vi "readFromXML.vi"(8 "error in (no error)":errorcluster, 10 "XMLin":string, 11 "RADecTarget in":refnum<class "RADecTarget.lvclass">) -> (0 "error out":errorcluster, 3 "RADecTarget out":refnum<class "RADecTarget.lvclass">)   [LabVIEW 2014, in "TCSDataDefinitions.lvlib" / "TCSCommand.lvlib" / "TargetConfiguration.lvlib" / "Target.lvlib" / "FixedTarget.lvlib" / "RADecTarget.lvclass"]
uses:
  RADecTarget.lvclass
  RADecTarget.lvclass/RADecTarget.ctl
  FixedTarget/FixedTarget.lvclass
  RADecParameters/RADecParameters.lvclass
  <userlib>/Common/XML/XMLParser/XMLParser.lvclass
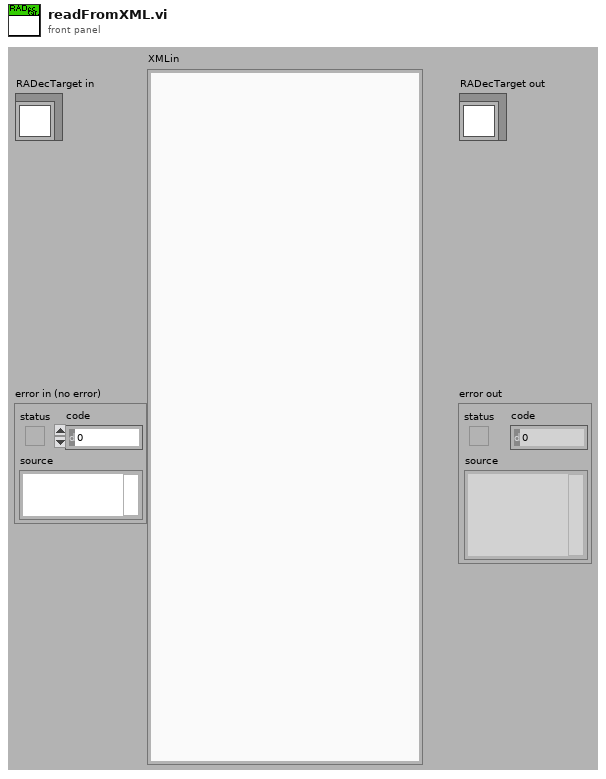
[diagram p1: front panel]
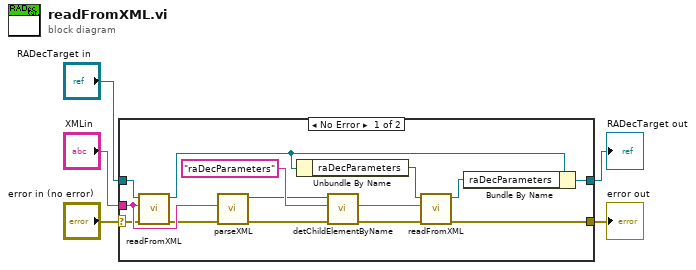
[diagram p0: block diagram]
diagram:
  n1 = case shown="No Error" "error in (no error)" {
    selector: "error in (no error)" -> [w9 w21]
    tunnel: [w12 w21] -> w4
    tunnel: [w14 w20] -> w2
    tunnel: "RADecTarget in" -> [w10 w20]
    tunnel: "XMLin" -> [w11 _]
    frame No Error {
      n2 = call-parent "readFromXML.vi"("error in (no error)"=w9, "XMLin"=w11, "FixedTarget in"=w10) -> ("error out"=w8:errorcluster, "FixedTarget out"=w7:refnum<class "RADecTarget.lvclass">)  [unwired: 7 in]
      n3 = call <userlib>:"parseXML.vi"("error in (no error)"=w8, "XMLString in"=w11) -> ("error out"=w19:errorcluster, "Element out"=w6:refnum<class "XMLParser.lvclass">)  [unwired: 8 in]
      n4 = Unbundle By Name(w7) -> ("raDecParameters"=w16:refnum<class "RADecParameters.lvclass">)
      n5 = call <userlib>:"detChildElementByName.vi"("error in (no error)"=w19, "childName"="raDecParameters" ("ChildName"), "Element in"=w6) -> ("error out"=w13:errorcluster, "childXML"=w17:string)  [unwired: 5 in, 2 out]
      n6 = call-dynamic "readFromXML.vi"("error in (no error)"=w13, "XMLin"=w17, "RADecParameters in"=w16) -> ("error out"=w12:errorcluster, "RADecParameters out"=w15:refnum<class "RADecParameters.lvclass">)  [unwired: 7 in]
      n7 = Bundle By Name(cluster=w7, "raDecParameters"=w15) -> (w14:refnum<class "RADecTarget.lvclass">)
    }
    frame Error {
    }
  }
  "error out" <- w4
  "RADecTarget out" <- w2
